vi "Set Signal Name.vi"(8 "error in (no error)":errorcluster, 10 "Step In":refnum<k7>, 11 "ModSweep in":refnum<class "ModSweep.lvclass">) -> (0 "error out":errorcluster, 2 "Step Out":refnum<k7>, 3 "ModSweep out":refnum<class "ModSweep.lvclass">)   [LabVIEW 2018, in "ModSweep.lvlib" / "ModSweep.lvclass"]
uses:
  ModSweep.lvclass
  Plugins/String Database.lvlibp/String Database.lvclass
  Plugins/TestStand API Tools (TSAT).lvlibp/Step Actions/TSAT Step Actions.lvlib
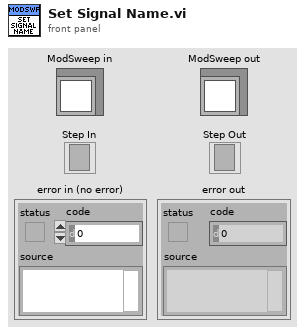
[diagram p1: front panel]
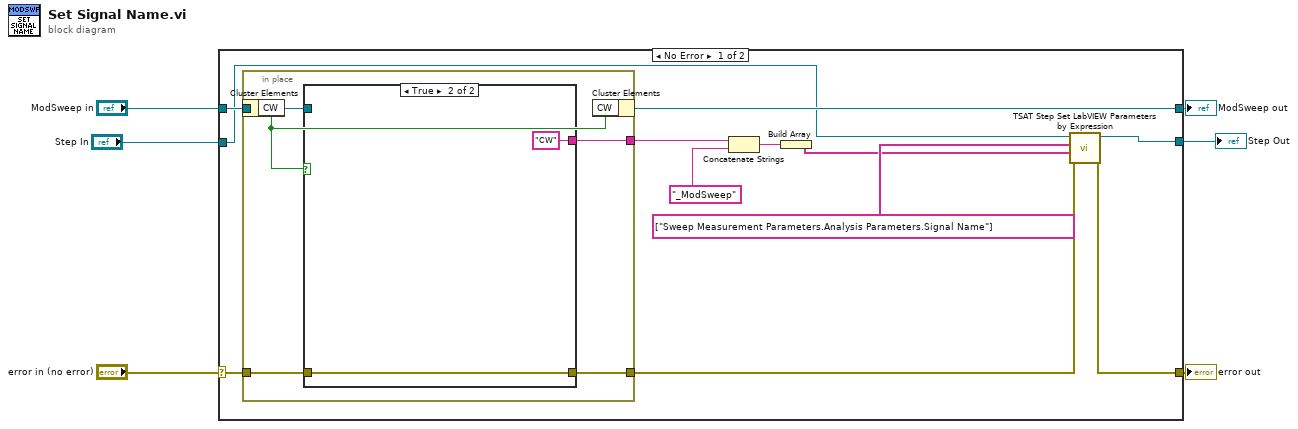
[diagram p0: block diagram]
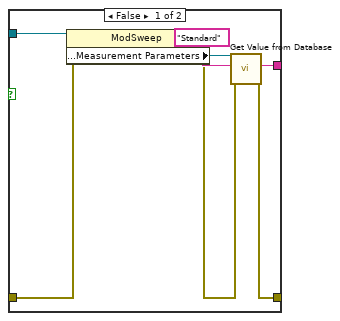
[diagram p2: hidden frame]
diagram:
  n1 = case shown="No Error" "error in (no error)" {
    selector: "error in (no error)" -> [w18 w35]
    tunnel: [w16 w35] -> w5
    tunnel: [w11 w34] -> w3
    tunnel: "ModSweep in" -> [w12 w34]
    tunnel: [w10 w33] -> w2
    tunnel: "Step In" -> [w9 w33]
    frame No Error {
      n2 = in-place {
        in-place-border: w18 -> [w23]
        in-place-border: w12 -> [w20]
        in-place-border: [w22] -> w17
        in-place-border: [w21] -> w15
        n3 = in-place-cluster #1(w12) -> ("CW"=w19:bool)
        n4 = case shown="True" w19 {
          tunnel: w23 -> [w30 w32]
          tunnel: [w27 w32] -> w22
          tunnel: [w26 "CW" ("Entry Value")] -> w21
          tunnel: w20 -> [w25 _]
          frame False {
            n5 = property class="ModSweep"(reference=w25, error in=w30) -> (error out=w24:errorcluster, "Protected Methods:Measurement Parameters"=w29:refnum<class "String Database.lvclass">)  [unwired: 1 out]
            n6 = call "Get Value from Database.vi"("error in (no error)"=w24, "Entry Name"="Standard", "Message in"=w29) -> ("error out"=w27:errorcluster, "Entry Value"=w26:string)  [unwired: 5 in, 2 out]
          }
          frame True {
          }
        }
        n7 = in-place-cluster #1("CW"=w19) -> (w11:refnum<class "ModSweep.lvclass">)
      }
      n8 = Concatenate Strings(w15, "_ModSweep" ("string")) -> (w13:string)
      n9 = Build Array(w13) -> (w7:string[])
      n10 = call "TSAT Step Set LabVIEW Parameters by Expression.vi"("Error In"=w17, "Value Expressions"=w7, "Parameters to Set"=string[] ["Sweep Measurement Parameters.Analysis Parameters.Signal Name"] ("Local Variable Mapping"), "Step In"=w9) -> ("Error Out"=w16:errorcluster, "Step Out"=w10:refnum<k7>)  [unwired: 6 in]
    }
    frame Error {
    }
  }
  "error out" <- w5
  "ModSweep out" <- w3
  "Step Out" <- w2
